vi "getValueChanged.vi"(8 "error in (no error)":errorcluster, 11 "Data in":refnum<class "Data.lvclass">) -> (0 "error out":errorcluster, 2 "Value Changed":refnum<user-event>, 3 "Data out":refnum<class "Data.lvclass">)   [LabVIEW 2017, in "Filled Text Fields.lvlib" / "Data.lvclass"]
uses:
  Data.lvclass
  Data.PrivateData.ctl
  Data.lvclass/Data.ctl
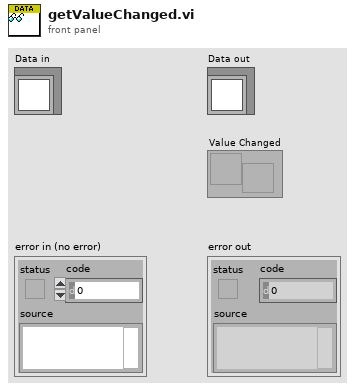
[diagram p1: front panel]
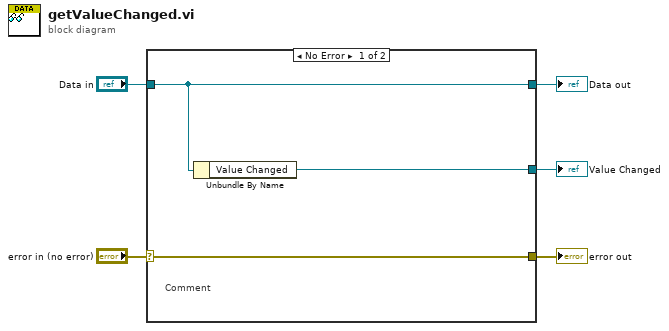
[diagram p0: block diagram]
diagram:
  n1 = case shown="No Error" "error in (no error)" {
    selector: "error in (no error)" -> [w8 w9]
    tunnel: [w8 w9] -> w4
    tunnel: [w7 w10] -> w2
    tunnel: "Data in" -> [w7 w10]
    tunnel: [w6 _] -> w1
    frame No Error {
      # "Comment"
      n2 = Unbundle By Name(w7) -> ("Value Changed"=w6:refnum<user-event>)
    }
    frame Error {
    }
  }
  "error out" <- w4
  "Data out" <- w2
  "Value Changed" <- w1
